vi "fChunk Counter.vi"(6 "Write mode":bool, 7 "Current File Number":i32, 8 "error In":errorcluster, 9 "Data Chunks per File":u32, 10 "Total Data Chunks to Write":dbl, 11 "Chunk In":u32) -> (0 "error out":errorcluster, 1 "File Writing Progress (%)":dbl(slide) scale=0.0..100.0, 3 "Chunk Out":u32)   [LabVIEW 2012]
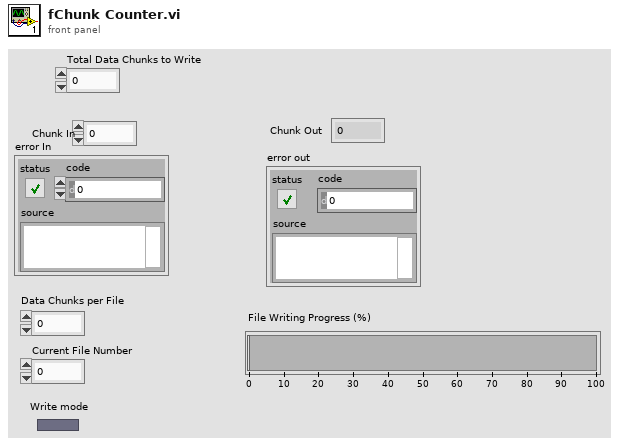
[diagram p1: front panel]
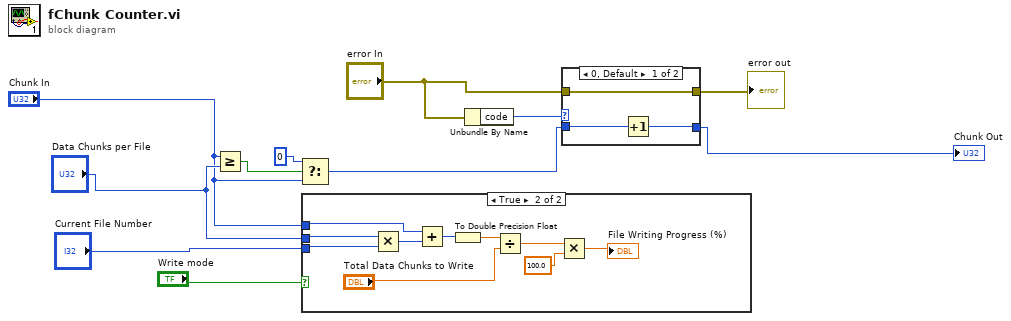
[diagram p0: block diagram]
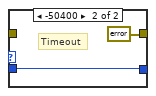
[diagram p2: hidden frame]
diagram:
  n1 = Greater Or Equal?(x="Chunk In", y="Data Chunks per File") -> (x >= y?=w10:bool)
  n2 = Select(t=u32 0, s=w10, f="Chunk In") -> (s? t:f=w5:u32)
  n3 = case shown="True" "Write mode" {
    tunnel: "Current File Number" -> [_ w21]
    tunnel: "Chunk In" -> [_ w19]
    tunnel: "Data Chunks per File" -> [_ w13]
    frame False {
    }
    frame True {
      n4 = Multiply(x=w13, y=w21) -> (x*y=w20:u32)
      n5 = Add(x=w19, y=w20) -> (x+y=w18:u32)
      n6 = To Double Precision Float(number=w18) -> (double precision float=w17:dbl)
      n7 = Divide(x=w17, y="Total Data Chunks to Write") -> (x/y=w15:dbl)
      n8 = Multiply(x=w15, y=100.0) -> (x*y=→"File Writing Progress (%)":dbl)
    }
  }
  n9 = Unbundle By Name("error In") -> ("code"=w1:i32)
  n10 = case shown="0, Default" w1 {
    tunnel: [w24 errorcluster {"status"=FALSE, "code"=0, "source"=""} ("error constant")] -> w7
    tunnel: "error In" -> [w24 _]
    tunnel: w5 -> [w23 w25]
    tunnel: [w22 w25] -> w4
    frame 0, Default {
      n11 = Increment(x=w23) -> (x+1=w22:u32)
    }
    frame -50400 {
      # "Timeout"
    }
  }
  "Chunk Out" <- w4
  "error out" <- w7
